vi "AImotive UDP Tester - Main.vi"(7 "destination address":string="localhost", 8 "error in":errorcluster, 9 "LabVIEW Tx port":u16=61556, 10 "LabVIEW Rx port":u16=61558, 11 "VeriStand Rx port":u16=61557) -> (0 "error out":errorcluster)   [LabVIEW 2019]
panel:
  out "*(type *) &x":string
  out "Rx Current Value":u8
  out "Tx Current Value":dbl
  in  "stop":bool
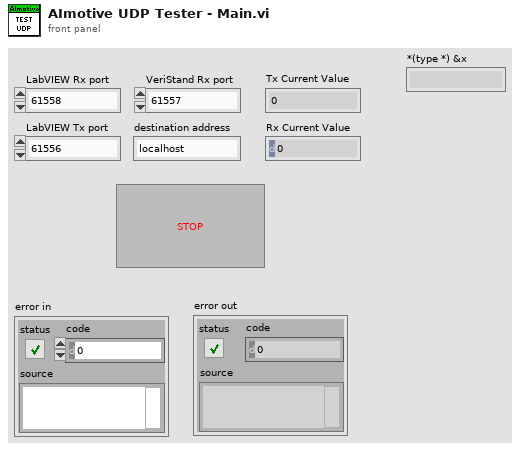
[diagram p1: front panel]
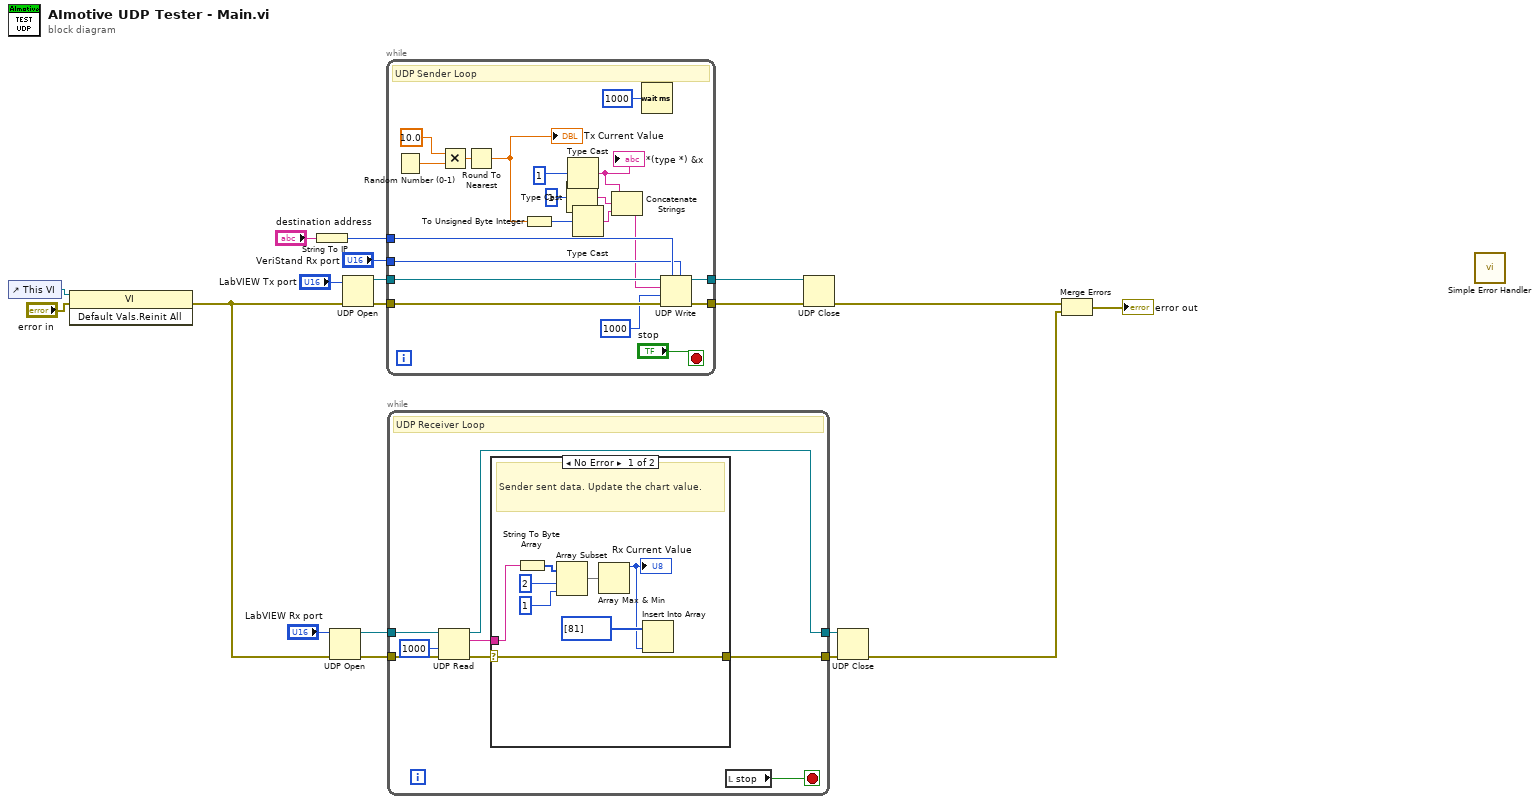
[diagram p0: block diagram]
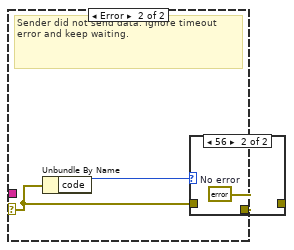
[diagram p2: hidden frame]
diagram:
  n1 = control-ref of="This VI"() -> (w3:refnum<vi>)
  n2 = invoke class="VI" method="Default Vals.Reinit All"(reference=w3, error in="error in") -> (error out=w1:errorcluster)  [unwired: 1 in, 2 out]
  n3 = String To IP(1:"destination address") -> (0:w15:u32)
  n4 = UDP Open(8:w1, 11:"LabVIEW Rx port") -> (port=w10:refnum<k16>, 0:w9:errorcluster)  [unwired: 3 in, 1 out]
  n5 = UDP Open(8:w1, 11:"LabVIEW Tx port") -> (port=w16:refnum<k16>, 0:w17:errorcluster)  [unwired: 3 in, 1 out]
  n6 = while {
    tunnel: [w34] -> w13
    tunnel: w16 -> [w39]
    tunnel: w17 -> [w38]
    tunnel: [w37] -> w12
    tunnel: w15 -> [w36]
    tunnel: "VeriStand Rx port" -> [w32]
    stop <- "stop" stop-if-true
    # "UDP Sender Loop"
    n7 = Random Number (0-1)() -> (number: 0 to 1=w30:dbl)
    n8 = Multiply(x=10.0, y=w30) -> (x*y=w28:dbl)
    n9 = Round To Nearest(number=w28) -> (nearest integer value=w26:dbl)
    "Tx Current Value" <- w26
    n10 = To Unsigned Byte Integer(number=w26) -> (unsigned 8bit integer=w25:u8)
    n11 = Type Cast(x=u32 1) -> (*(type *) &x=w22:string)  [unwired: 1 in]
    n12 = Type Cast(x=u16 1) -> (*(type *) &x=w24:string)  [unwired: 1 in]
    "*(type *) &x" <- w24
    n13 = Type Cast(x=w25) -> (*(type *) &x=w23:string)  [unwired: 1 in]
    n14 = Concatenate Strings(w24, w22, w23) -> (w27:string)
    n15 = Wait (ms)(milliseconds to wait=u32 1000) -> ()  [unwired: 1 out]
    n16 = UDP Write(address=w36, port or service name=w32, connection ID=w39, data in=w27, 8:w38, 9:1000 ("timeout ms (25000)")) -> (error out=w34:errorcluster, 3:w37:refnum<k16>)
  }
  n17 = while {
    tunnel: w10 -> [w47]
    tunnel: [w42] -> w7
    tunnel: w9 -> [w46]
    tunnel: [w43] -> w8
    stop <- w41 stop-if-true
    # "UDP Receiver Loop"
    n18 = UDP Read(connection ID=w47, timeout ms (25000)=1000, 8:w46) -> (data out=w45:string, error out=w44:errorcluster, 3:w42:refnum<k16>)  [unwired: 3 out]
    n19 = case shown="No Error" w44 {
      selector: w44 -> [w55 w57]
      tunnel: w45 -> [w53 _]
      tunnel: [w55 w56] -> w43
      frame No Error {
        # "Sender sent data. Update the chart value."
        n20 = String To Byte Array(string=w53) -> (unsigned byte array=w54:u8[])
        n21 = Array Subset(array=w54, index=2 ("length"), length=1) -> (w50:u8[])
        n22 = Array Max & Min(array=w50) -> (max value=w48:u8)  [unwired: 3 out]
        "Rx Current Value" <- w48
        n23 = Insert Into Array(array=u8[] [81] ("Rx Array"), new element=w48) -> ()  [unwired: 1 in, 1 out]
      }
      frame Error {
        (unwired) u8 0
        # "Sender did not send data. Ignore timeout error and keep waiting."
        n24 = Unbundle By Name(w57) -> ("code"=w58:i32)
        n25 = case shown="56" w58 {
          tunnel: w57 -> [w59 _]
          tunnel: [w59 w60] -> w56
          frame Default {
          }
          frame 56 {
            w60 = errorcluster {"status"=FALSE, "code"=0, "source"=""}  # No error
          }
        }
      }
    }
    n26 = local read "stop"() -> (w41:bool)
  }
  n27 = UDP Close(connection ID=w12, 8:w13) -> (error out=w6:errorcluster)  [unwired: 1 out]
  n28 = UDP Close(connection ID=w7, 8:w8) -> (error out=w4:errorcluster)  [unwired: 1 out]
  n29 = Merge Errors(w6, w4) -> (→"error out":errorcluster)
  n30 = call <vilib>:"Simple Error Handler.vi"() -> ()  [unwired: 5 in, 5 out]
